vi "VI-Replace Objects in Factory.vi"(7 "vi path":path, 11 "error in (no error)":errorcluster, 12 "by name":path) -> (15 "error out":errorcluster)   [LabVIEW 2020]
uses:
  <vilib>/Utility/traverseref.llb/TRef TravTarget.ctl
  <vilib>/Utility/traverseref.llb/VI Scripting - Traverse.lvlib
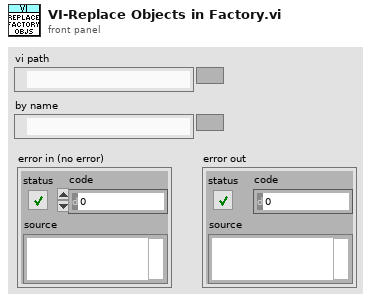
[diagram p1: front panel]
types:
  T1 = typedef "TRef TravTarget.ctl" = enum16{"FP", "BD", "Other"}
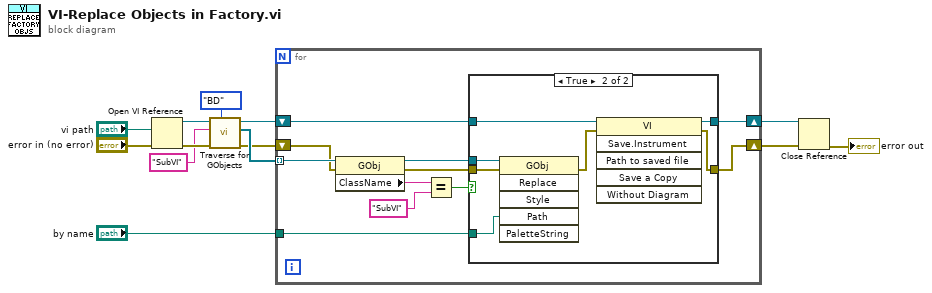
[diagram p0: block diagram]
diagram:
  n1 = Open VI Reference(vi path="vi path", error in (no error)="error in (no error)") -> (vi reference=w13:refnum<vi>, error out=w12:errorcluster)  [unwired: 4 in]
  n2 = call <vilib>:"Traverse for GObjects.vi"("Traverse Target"=TRef_TravTarget."BD", "error in (no error)"=w12, "Class Name"="SubVI", "VI Refnum"=w13) -> ("error out"=w8:errorcluster, "References"=w9:refnum<vi>[], "dup VI Refnum"=w6:refnum<vi>)  [unwired: 4 in, 1 out]
  n3 = for {
    tunnel: w9 -> [w24] mode=indexing
    shift-right: [w18] -> w3
    shift-left: w8 -> [w23]
    shift-right: [w16] -> w4
    shift-left: w6 -> [w17]
    tunnel: "by name" -> [w15]
    n4 = property class="GObj"(reference=w24, error in=w23) -> (reference out=w21:refnum<vi>, error out=w19:errorcluster, "ClassName"=w14:string)
    n5 = Equal?(x=w14, y="SubVI") -> (x = y?=w20:bool)
    n6 = case shown="True" w20 {
      tunnel: w21 -> [_ w33]
      tunnel: w19 -> [w26 w32]
      tunnel: [w26 w29] -> w18
      tunnel: w17 -> [w25 w31]
      tunnel: [w25 w28] -> w16
      tunnel: w15 -> [_ w27]
      frame False {
      }
      frame True {
        n7 = invoke class="GObj" method="Replace"(reference=w33, error in=w32, "Path"=w27) -> (error out=w30:errorcluster)  [unwired: 3 in, 5 out]
        n8 = invoke class="VI" method="Save.Instrument"(reference=w31, error in=w30) -> (reference out=w28:refnum<vi>, error out=w29:errorcluster)  [unwired: 4 in, 4 out]
      }
    }
  }
  n9 = Close Reference(reference=w4, error in (no error)=w3) -> (error out=→"error out":errorcluster)
